vi "ATF-CS- Queue Data log module.vi"(8 "error in":errorcluster, 11 "?":T1) -> (0 "error out":errorcluster)   [LabVIEW 2022 SP3]
uses:
  UI Message handler/Message Queue/All Message Queues.ctl
  UI Message handler/Message Queue/Message Cluster.ctl
  Controls/SeCrTs-CS Datalog enum.ctl
  UI Message handler/Message Queue/Message Queue.lvlib
panel:
  out "Log health":bool
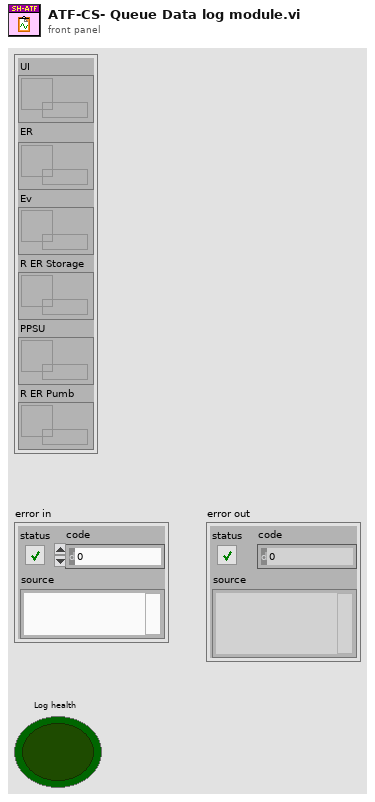
[diagram p1: front panel]
types:
  T1 = typedef "Message Queue.lvlib/All Message Queues.ctl" = cluster{"UI":refnum<queue>, "ER":refnum<queue>, "Ev":refnum<queue>, "R ER Storage":refnum<queue>, "PPSU":refnum<queue>, "R ER Pumb":refnum<queue>}
  T2 = cluster{"Log In Progress?":bool, "Log Start Time":timestamp, "Analog Queues":refnum<queue>[], "Digital Queues":refnum<queue>[], "tdms file ref":refnum<k34>}
  T3 = typedef "SeCrTs-CS Datalog enum.ctl" = enum16{"Initialize", "Poll", "Create file", "log Analog", "log Digital", "Flush Queues", "Close file", "Error", "Exit"}
  T4 = enum16{"open", "open or create", "create or replace", "create", "open (read-only)"}
  T5 = typedef "SeCrTs-file folder ctl.ctl" = cluster{"Datalog path":path, "Configuration path":path, "Signal list path":path, "Sub vi's":path, "Authentication":path, "Sequence":path, "Event Log":path, "CS Error log":path, "RT Error Log":path}
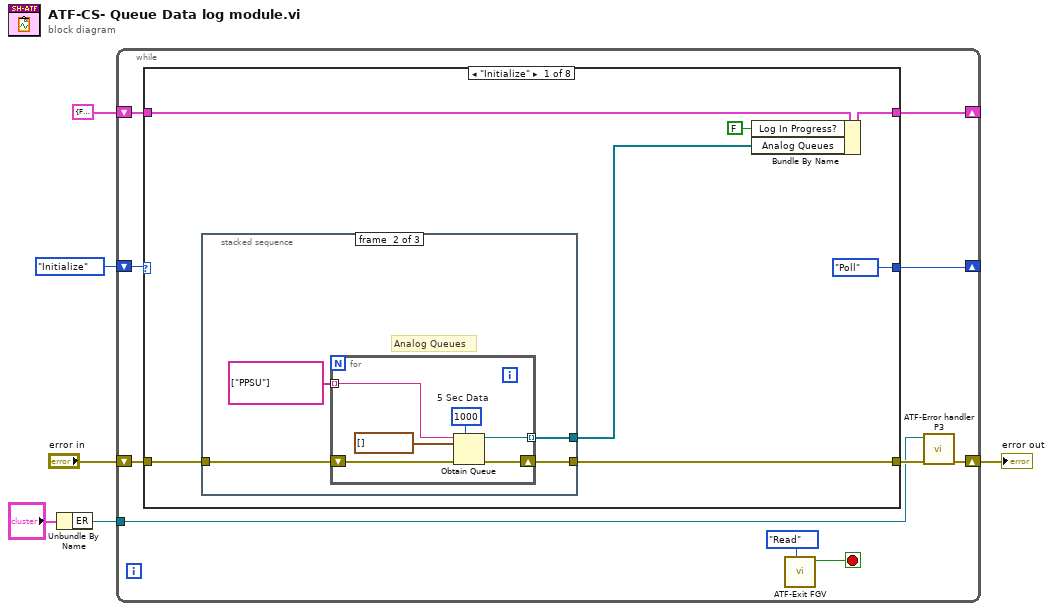
[diagram p0: block diagram]
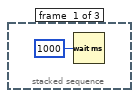
[diagram p2: hidden frame]
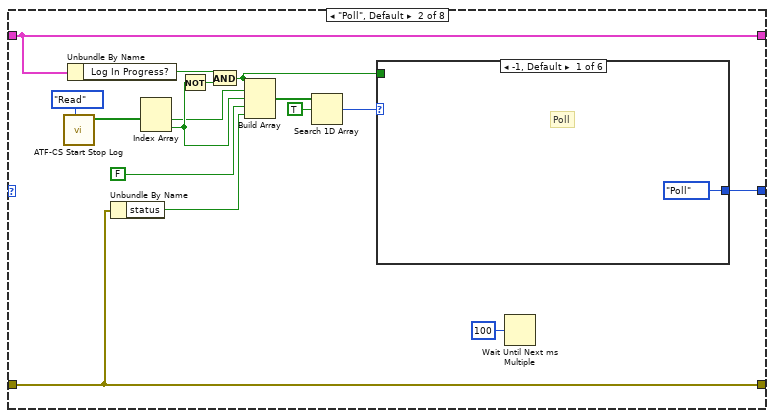
[diagram p4: hidden frame]
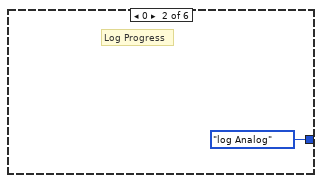
[diagram p5: hidden frame]
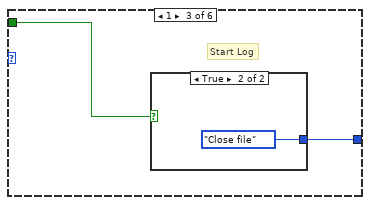
[diagram p6: hidden frame]
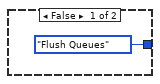
[diagram p7: hidden frame]
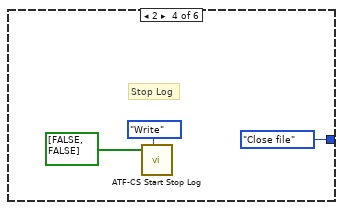
[diagram p8: hidden frame]
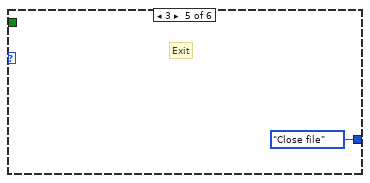
[diagram p9: hidden frame]
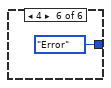
[diagram p10: hidden frame]
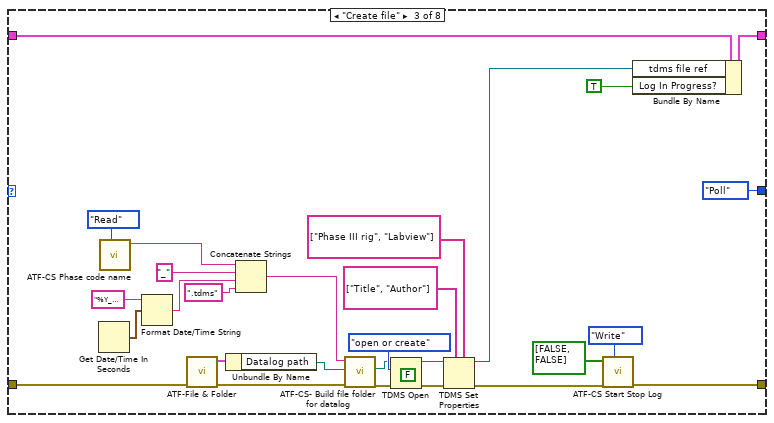
[diagram p11: hidden frame]
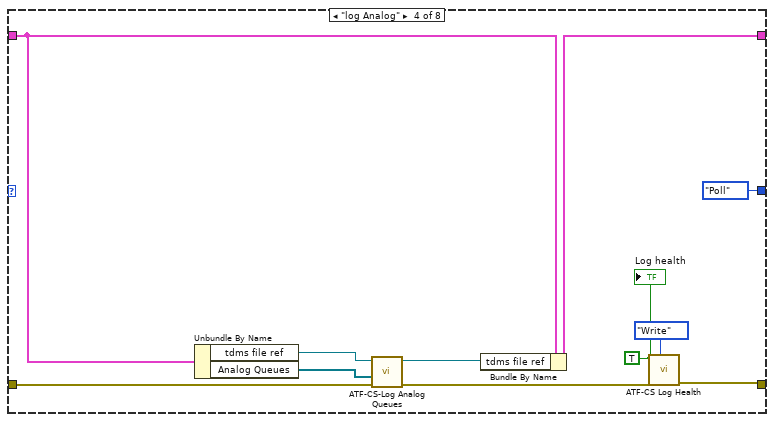
[diagram p12: hidden frame]
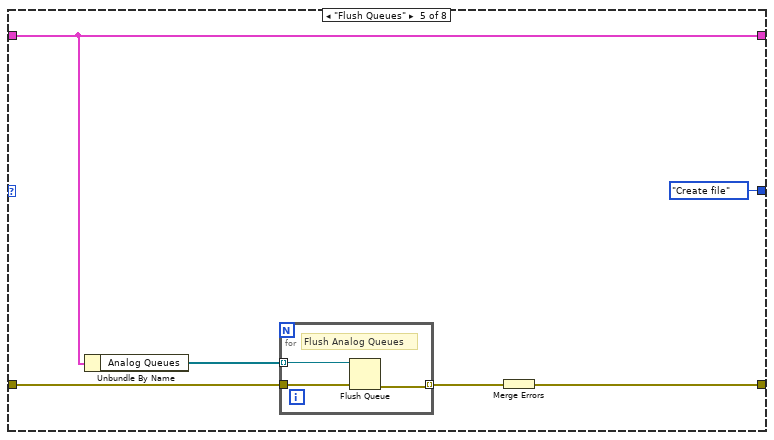
[diagram p13: hidden frame]
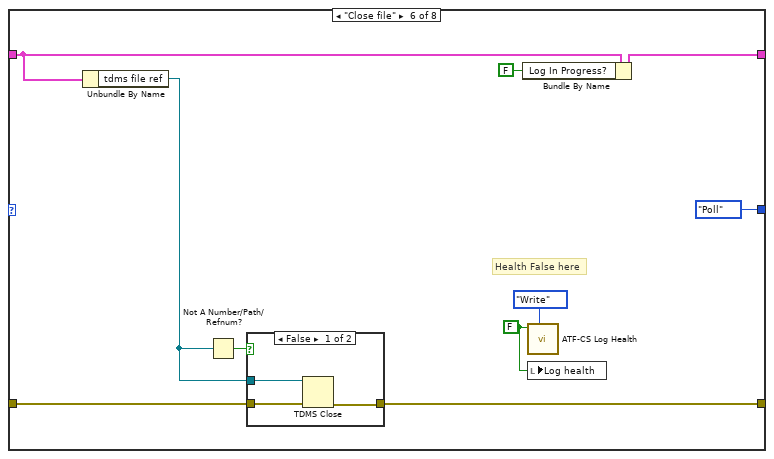
[diagram p14: hidden frame]
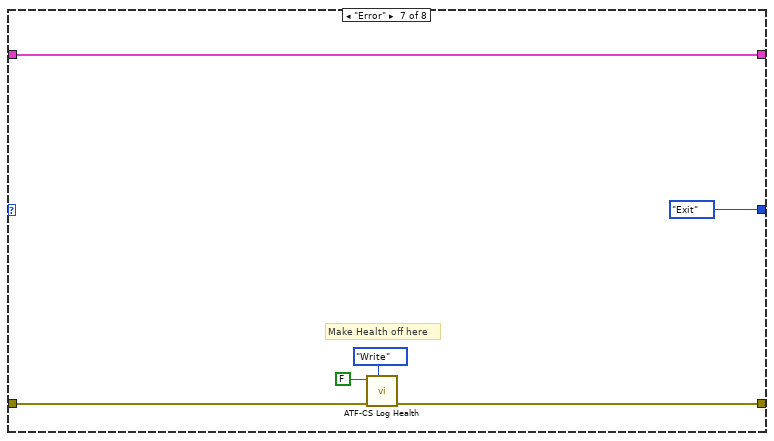
[diagram p16: hidden frame]
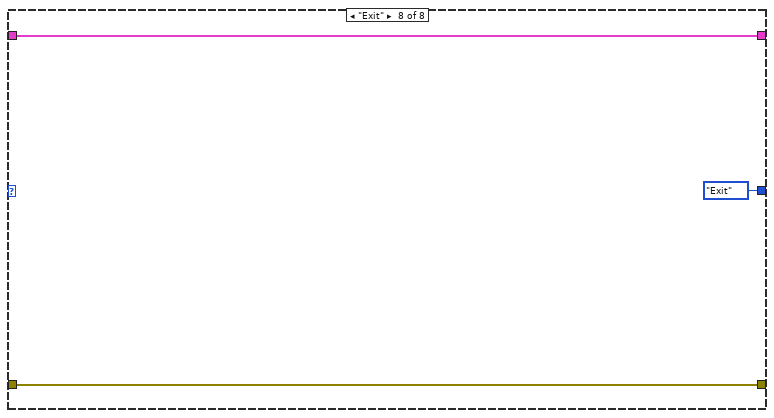
[diagram p17: hidden frame]
diagram:
  n1 = Unbundle By Name("?") -> ("ER"=w1:refnum<queue>)
  n2 = while {
    shift-right: [w12] -> _
    shift-left: SeCrTs-CS_Datalog_enum."Initialize" -> [w16]
    shift-right: [w13] -> _
    shift-left: T2 {"Log In Progress?"=FALSE, "Log Start Time"=timestamp(0 s since 1904-01-01), "Analog Queues"=[], "Digital Queues"=[], "tdms file ref"=refnum} -> [w14]
    shift-right: [w8] -> w3
    shift-left: "error in" -> [w15]
    tunnel: w1 -> [w7]
    stop <- w10 stop-if-true
    n3 = case shown="\"Initialize\"" w16 {
      tunnel: w15 -> [w22 w44 w83 w97 w103 w115 w125 w131]
      tunnel: w14 -> [w23 w50 w72 w99 w105 w116 w129 w132]
      tunnel: [w21 w50 w71 w95 w105 w118 w129 w132] -> w13
      tunnel: [w18 w44 w62 w90 w101 w114 w124 w131] -> w9
      tunnel: [SeCrTs-CS_Datalog_enum."Poll" w45 SeCrTs-CS_Datalog_enum."Poll" SeCrTs-CS_Datalog_enum."Poll" SeCrTs-CS_Datalog_enum."Create file" SeCrTs-CS_Datalog_enum."Poll" SeCrTs-CS_Datalog_enum."Exit" SeCrTs-CS_Datalog_enum."Exit"] -> w12
      frame "Initialize" {
        n4 = stacked-sequence {
          tunnel: w22 -> [_ w27 _]
          tunnel: [_ w28 _] -> w19
          tunnel: [_ w26 _] -> w18
          frame #0 {
            n5 = Wait (ms)(milliseconds to wait=u32 1000) -> ()  [unwired: 1 out]
          }
          frame #1 {
            # "Analog Queues"
            n6 = for {
              tunnel: [w31] -> w28 mode=indexing
              shift-right: [w33] -> w26
              shift-left: w27 -> [w34]
              tunnel: string[] ["PPSU"] ("Array") -> [w30] mode=indexing
              w32 = 1000  # 5 Sec Data
              n7 = Obtain Queue(max queue size (-1, unlimited)=w32, name (unnamed)=w30, element data type=waveform(dbl)[] [] ("data"), error in (no error)=w34) -> (queue out=w31:refnum<queue>, error out=w33:errorcluster)  [unwired: 1 in, 1 out]
            }
          }
          frame #2 {
            # "Datalog loop running Status"
          }
        }
        n8 = Bundle By Name(cluster=w23, "Log In Progress?"=FALSE, "Analog Queues"=w19) -> (w21:T2)
      }
      frame "Poll", Default {
        n9 = call "ATF-CS Start Stop Log.vi"("Enum"=enum16{"Read", "Write"}."Read") -> ("Start Stop log R"=w38:bool[])  [unwired: 9 in, 1 out]
        n10 = Unbundle By Name(w50) -> ("Log In Progress?"=w43:bool)
        n11 = Unbundle By Name(w44) -> ("status"=w49:bool)
        n12 = Index Array(array=w38) -> (element #1=w40:bool, element #2=w41:bool)  [unwired: 2 in]
        n13 = Not(x=w41) -> (.not. x?=w42:bool)
        n14 = And(x=w43, y=w42) -> (x .and. y?=w37:bool)
        n15 = Build Array(w37, w40, w41, FALSE, w49) -> (w48:bool[])
        n16 = Search 1D Array(1D array=w48, element=TRUE) -> (index of element=w46:i32)  [unwired: 1 in]
        n17 = case shown="-1, Default" w46 {
          tunnel: [SeCrTs-CS_Datalog_enum."Poll" SeCrTs-CS_Datalog_enum."log Analog" w54 SeCrTs-CS_Datalog_enum."Close file" SeCrTs-CS_Datalog_enum."Close file" SeCrTs-CS_Datalog_enum."Error"] -> w45
          tunnel: w37 -> [_ _ w53 _ _ _]
          frame -1, Default {
            # "Poll"
          }
          frame 0 {
            # "Log Progress"
          }
          frame 1 {
            # "Start Log"
            n18 = case shown="True" w53 {
              tunnel: [SeCrTs-CS_Datalog_enum."Flush Queues" SeCrTs-CS_Datalog_enum."Close file"] -> w54
              frame False {
              }
              frame True {
              }
            }
          }
          frame 2 {
            # "Stop Log"
            n19 = call "ATF-CS Start Stop Log.vi"("Enum"=enum16{"Read", "Write"}."Write", "Start Stop log"=bool[] [FALSE, FALSE]) -> ()  [unwired: 8 in, 2 out]
          }
          frame 3 {
            # "Exit"
          }
          frame 4 {
          }
        }
        n20 = Wait Until Next ms Multiple(millisecond multiple=u32 100) -> ()  [unwired: 1 out]
      }
      frame "Create file" {
        (unwired) FALSE ("disable buffering? (T)")
        n21 = Get Date/Time In Seconds() -> (seconds since 1Jan1904=w85:timestamp)
        n22 = call "ATF-CS Phase code name.vi"("Enum"=enum16{"Read", "Write"}."Read") -> ("Phase codeR"=w64:string)  [unwired: 9 in, 1 out]
        n23 = Format Date/Time String(time format string (%c)="%Y_%b_%d_%Hh_%Mm_%Ssec", seconds (now)=w85) -> (date/time string=w89:string)  [unwired: 1 in]
        n24 = call "ATF-File & Folder.vi"("error in (no error)"=w83) -> ("error out"=w82:errorcluster, "File Output"=w81:T5)  [unwired: 9 in]
        n25 = Unbundle By Name(w81) -> ("Datalog path"=w80:path)
        n26 = Concatenate Strings(w64, "_" ("string"), w89, ".tdms" ("string")) -> (w84:string)
        n27 = call "ATF-CS- Build file folder for datalog.vi"("error in (no error)"=w82, "Base Path"=w80, "File Name"=w84) -> ("error out"=w74:errorcluster, "Result File path"=w73:path)  [unwired: 6 in, 1 out]
        n28 = TDMS Open(8:w74, 10:T4."open or create" ("operation (0:open)"), 11:w73) -> (0:w78:errorcluster, 3:w77:refnum<k34>)  [unwired: 4 in]
        n29 = TDMS Set Properties(5:string[] ["Phase III rig", "Labview"] ("property names"), 7:string[] ["Title", "Author"] ("property names"), 8:w78, 11:w77) -> (0:w63:errorcluster, 3:w70:refnum<k34>)  [unwired: 4 out]
        n30 = call "ATF-CS Start Stop Log.vi"("Enum"=enum16{"Read", "Write"}."Write", "error in"=w63, "Start Stop log"=bool[] [FALSE, FALSE]) -> ("error out"=w62:errorcluster)  [unwired: 7 in, 1 out]
        n31 = Bundle By Name(cluster=w72, "tdms file ref"=w70, "Log In Progress?"=TRUE) -> (w71:T2)
      }
      frame "log Analog" {
        w92 = TRUE ("Log health")
        n32 = Unbundle By Name(w99) -> ("tdms file ref"=w96:refnum<k34>, "Analog Queues"=w98:refnum<queue>[])
        n33 = call "ATF-CS-Log Analog Queues.vi"("error in"=w97, "Analog queues"=w98, "tdms file in"=w96) -> ("error out"=w91:errorcluster, "tdms ref out"=w94:refnum<k34>)  [unwired: 7 in]
        n34 = Bundle By Name(cluster=w99, "tdms file ref"=w94) -> (w95:T2)
        n35 = call "ATF-CS Log Health.vi"("Enum"=enum16{"Read", "Write"}."Write", "error in"=w91, "Log health"=w92) -> ("error out"=w90:errorcluster)  [unwired: 7 in, 1 out]
        "Log health" <- w92
      }
      frame "Flush Queues" {
        n36 = Unbundle By Name(w105) -> ("Analog Queues"=w104:refnum<queue>[])
        n37 = for {
          tunnel: w104 -> [w109] mode=indexing
          tunnel: w103 -> [w108]
          tunnel: [w107] -> w102 mode=indexing
          # "Flush Analog Queues"
          n38 = Flush Queue(queue=w109, error in (no error)=w108) -> (error out=w107:errorcluster)  [unwired: 2 out]
        }
        n39 = Merge Errors(w102) -> (w101:errorcluster)
      }
      frame "Close file" {
        w110 = FALSE ("Log health")
        # "Health False here"
        n40 = Unbundle By Name(w116) -> ("tdms file ref"=w112:refnum<k34>)
        n41 = Not A Number/Path/Refnum?(number/path/refnum=w112) -> (NaN/Path/Refnum?=w113:bool)
        n42 = case shown="False" w113 {
          tunnel: w115 -> [w122 w123]
          tunnel: [w121 w123] -> w114
          tunnel: w112 -> [w120 _]
          frame False {
            n43 = TDMS Close(8:w122, 11:w120) -> (0:w121:errorcluster)  [unwired: 1 out]
          }
          frame True {
          }
        }
        n44 = Bundle By Name(cluster=w116, "Log In Progress?"=FALSE) -> (w118:T2)
        n45 = call "ATF-CS Log Health.vi"("Enum"=enum16{"Read", "Write"}."Write", "Log health"=w110) -> ()  [unwired: 8 in, 2 out]
        n46 = local write "Log health"(w110) -> ()
      }
      frame "Error" {
        # "Make Health off here"
        n47 = call "ATF-CS Log Health.vi"("Enum"=enum16{"Read", "Write"}."Write", "error in"=w125, "Log health"=FALSE) -> ("error out"=w124:errorcluster)  [unwired: 7 in, 1 out]
      }
      frame "Exit" {
      }
    }
    n48 = call "ATF-Exit FGV.vi"("Enum"=enum16{"Init", "Read", "Write"}."Read") -> ("Exit R"=w10:bool)  [unwired: 9 in, 1 out]
    n49 = call "ATF-Error handler P3.vi"("error in"=w9, "Message Queue"=w7) -> ("error out"=w8:errorcluster)  [unwired: 8 in, 1 out]
  }
  "error out" <- w3
